vi "AT Set Bool A.vi"(8 "error in (no error)":errorcluster, 9 "Value":bool, 10 "Feature":string, 11 "Handle":i32) -> (0 "error out":errorcluster, 3 "Status":i32)   [LabVIEW 2009]
doc: "Set Bool\n\nOutput:\n I32 Status\n\nInput:\n I32 Handle\n String Feature\n Bool Value\n\nThis function will set the value of the specified boolean feature. A value of FALSE indicates false and a\nvalue of TRUE indicates true. An error will be returned if the feature is read only, currently not writable, not a boolean feature or is not implemented by the camera."
uses:
  atcoreA.dll
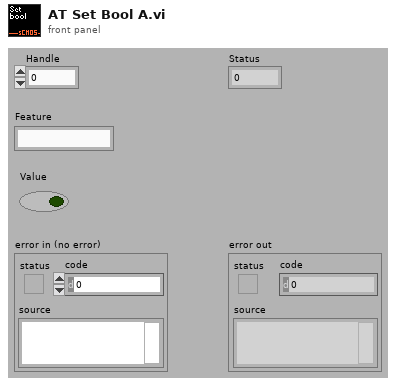
[diagram p1: front panel]
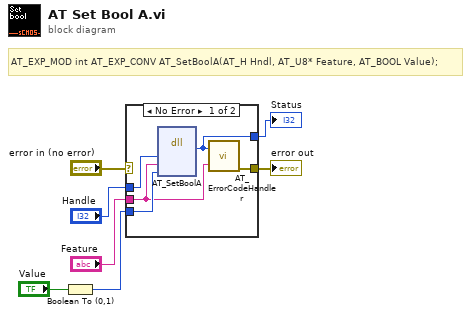
[diagram p0: block diagram]
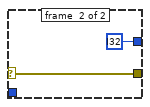
[diagram p2: hidden frame]
diagram:
  # "AT_EXP_MOD int AT_EXP_CONV AT_SetBoolA(AT_H Hndl, AT_U8* Feature, AT_BOOL Value);"
  n1 = Boolean To (0,1)(Boolean="Value") -> (0, 1=w3:i16)
  n2 = case shown="No Error" "error in (no error)" {
    selector: "error in (no error)" -> [_ w14]
    tunnel: [w9 i32 ? ("Status")] -> w7
    tunnel: "Handle" -> [w12 _]
    tunnel: "Feature" -> [w8 _]
    tunnel: w3 -> [w11 _]
    tunnel: [w10 w14] -> w1
    frame #0 {
      n3 = dll-call lib="atcoreA.dll" fn="AT_SetBoolA"("Handle"=w12, "Feature"=w8, "Value"=w11) -> ("Status"=w9:i32)  [unwired: 6 in, 2 out]
      n4 = call "AT_ErrorCodeHandler.vi"("Error"=w9, "Feature Name"=w8) -> ("error out"=w10:errorcluster)  [unwired: 5 in]
    }
    frame #1 {
    }
  }
  "Status" <- w7
  "error out" <- w1
